vi "Station Get By IP.vi"(8 "error in (no error)":errorcluster, 10 "IP or Name (\"\")":string, 11 "Connection Refnum":T3) -> (0 "error out":errorcluster, 1 "Instruments on Station":T2[](array[typedef]), 2 "Station Record":T1, 3 "Connection Refnum":T3, 4 "Data Present?":bool, 6 "Stand Alone?":bool)   [LabVIEW 2011]
uses:
  SI.LIB/ODBC/SQL Controls/Connection Refnum.ctl
  Instruments/Instrument Record.ctl
  Station Record.ctl
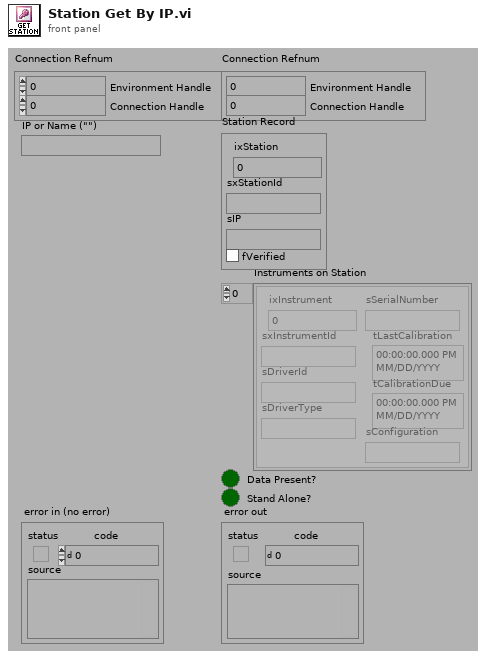
[diagram p1: front panel]
types:
  T1 = typedef "Station Record.ctl" = cluster{"ixStation":i32, "sxStationId":string, "sIP":string, "fVerified":bool}
  T2 = typedef "Instrument Record.ctl" = cluster{"ixInstrument":i32, "sxInstrumentId":string, "sDriverId":string, "sDriverType":string, "sSerialNumber":string, "tLastCalibration":timestamp, "tCalibrationDue":timestamp, "sConfiguration":string}
  T3 = typedef "Connection Refnum.ctl" = cluster{"Environment Handle":i32, "Connection Handle":i32}
  T4 = typedef "Statement Refnum.ctl" = cluster{"Statement Handle":i32, "Parameter Number":u16}
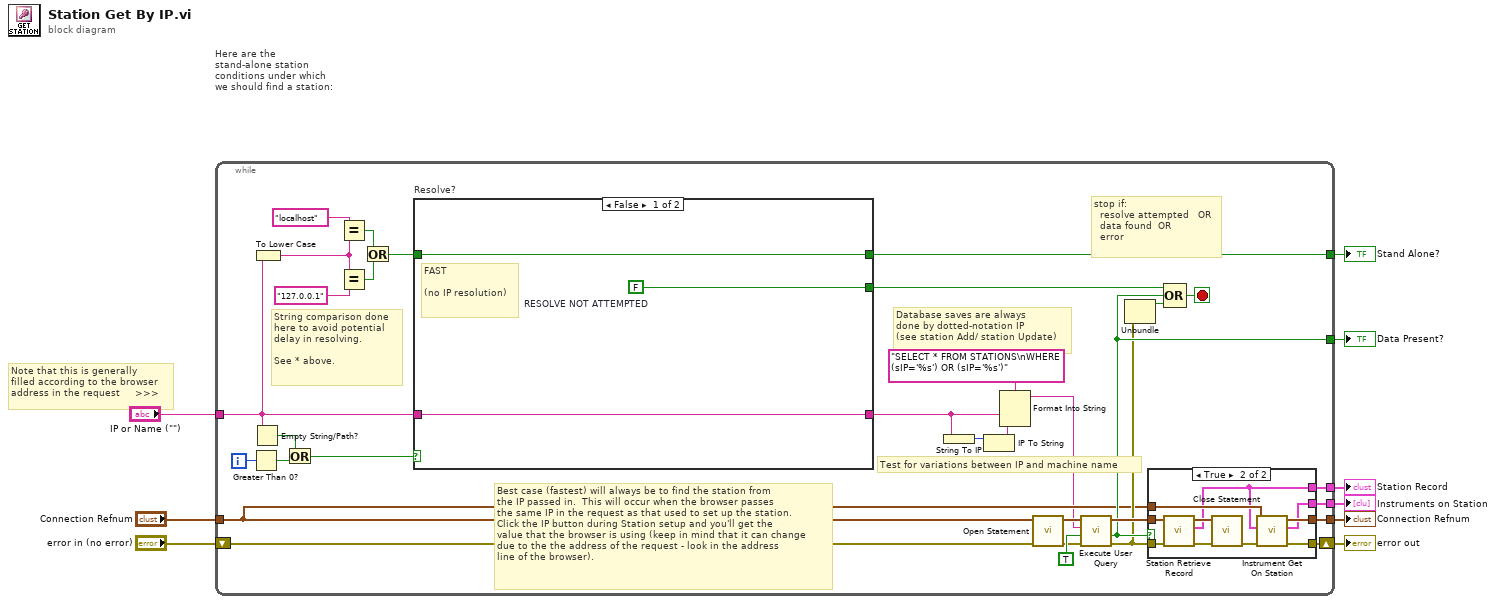
[diagram p0: block diagram]
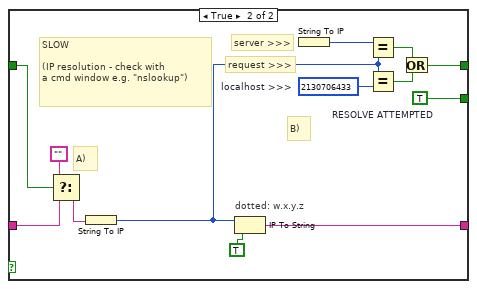
[diagram p2: hidden frame]
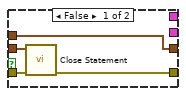
[diagram p3: hidden frame]
diagram:
  # "Note that this is generally\nfilled according to the browser\naddress in the request     >>>"
  n1 = while "Here are the stand-alone station conditions under which we should find a station:\n\n    1) Station saved by \"real\" IP (or domain name);  Request is from 127.0.0.1 (or localhost)\n    2) Station saved by \"127.0.0.1\" or (localhost);  Request from \"real\" IP (or domain name)\n---------------\n0 (fast).  Try query by incoming IP (or Name) without resolving    \n1 (slow).  If not found, try resolving incoming IP, then query.\n                a)  if incoming is \"localhost\" or \"127.0.0.1\" then force to empty \"\" as we've\n                     already looked for these in the first pass;\n                b) if incoming is NOT localhost IP, try to resolve, and compare resolved IP (numeric)\n                    with the server's IP to get \"stand-alone\" status." {
    tunnel: [w38] -> w9
    tunnel: "Connection Refnum" -> [w26]
    tunnel: "IP or Name (\"\")" -> [w17]
    tunnel: [w25] -> w5
    shift-right: [w27] -> w6
    shift-left: "error in (no error)" -> [w33]
    tunnel: [w13] -> w7
    tunnel: [w12] -> w4
    tunnel: [w11] -> w3
    i -> [w39]
    stop <- w37 stop-if-true
    # "Test for variations between IP and machine name"
    # "String comparison done\nhere to avoid potential\ndelay in resolving. \n\nSee * above."
    # "Database saves are always\ndone by dotted-notation IP\n(see station Add/ station Update)"
    # "Best case (fastest) will always be to find the station from\nthe IP passed in.  This will occur when the browser passes\nthe same IP in the request as that used to set up the station.\nClick the IP button during Station setup and you'll get the\nvalue that the browser is using (keep in mind that it can change\ndue to the the address of the request - look in the address\nline of the browser)."
    # "stop if:\n  resolve attempted   OR\n  data found  OR\n  error"
    n2 = Greater Than 0?(x=w39) -> (x > 0?=w29:bool)
    n3 = Empty String/Path?(string/path=w17) -> (empty?=w30:bool)
    n4 = To Lower Case(string=w17) -> (all lower case string=w18:string)
    n5 = Or(x=w30, y=w29) -> (x .or. y?=w28:bool)
    n6 = Equal?(x="localhost", y=w18) -> (x = y?=w21:bool)
    n7 = Equal?(x=w18, y="127.0.0.1") -> (x = y?=w22:bool)
    n8 = Or(x=w21, y=w22) -> (x .or. y?=w16:bool)
    n9 = case "Resolve?" shown="False" w28 {
      tunnel: [w43 w57] -> w10
      tunnel: w17 -> [w43 w54]
      tunnel: [w44 w45] -> w31
      tunnel: [w42 w46] -> w13
      tunnel: w16 -> [w42 w55]
      frame False {
        w44 = FALSE  # RESOLVE NOT ATTEMPTED
        # "FAST\n\n(no IP resolution)"
      }
      frame True {
        w45 = TRUE  # RESOLVE ATTEMPTED
        w49 = u32 2130706433  # localhost >>>
        # "B)"
        # "request >>>"
        # "server >>>"
        # "A)"
        # "SLOW\n\n(IP resolution - check with\na cmd window e.g. \"nslookup\")"
        # "dotted: w.x.y.z"
        n10 = Select(t="", s=w55, f=w54) -> (s? t:f=w53:string)
        n11 = String To IP(1:w53) -> (0:w47:u32)
        n12 = IP To String(1:TRUE, 2:w47) -> (0:w57:string)
        n13 = String To IP() -> (0:w51:u32)  [unwired: 1 out]
        n14 = Equal?(x=w51, y=w47) -> (x = y?=w50:bool)
        n15 = Equal?(x=w47, y=w49) -> (x = y?=w48:bool)
        n16 = Or(x=w50, y=w48) -> (x .or. y?=w46:bool)
      }
    }
    n17 = String To IP(1:w10) -> (0:w15:u32)
    n18 = IP To String(2:w15) -> (0:w14:string)  [unwired: 1 out]
    n19 = Format Into String(format string="SELECT * FROM STATIONS\nWHERE (sIP='%s') OR (sIP='%s')" ("User Query"), w10, w14) -> (resulting string=w23:string)  [unwired: 2 in, 1 out]
    n20 = call "Open Statement.vi"("error in (no error)"=w33, "Connection Refnum"=w26) -> ("error out"=w32:errorcluster, "Statement Refnum"=w34:T4)  [unwired: 4 out]
    n21 = call "Execute User Query.vi"("error in (no error)"=w32, "Return Data? (f)"=TRUE, "User Query"=w23, "Statement Refnum"=w34) -> ("error out"=w36:errorcluster, "Data Present?"=w38:bool, "Statement Refnum"=w41:T4)  [unwired: 1 out]
    n22 = Unbundle(w36) -> ("status"=w35:bool)  [unwired: 2 out]
    n23 = case shown="True" w38 {
      tunnel: w36 -> [w61 w71]
      tunnel: w41 -> [w60 w70]
      tunnel: [w59 w66] -> w27
      tunnel: w26 -> [w58 w65]
      tunnel: [w58 w64] -> w25
      tunnel: [_ w63] -> w12
      tunnel: [_ w62] -> w11
      frame False {
        n24 = call "Close Statement.vi"("error in (no error)"=w61, "Statement Refnum"=w60) -> ("error out"=w59:errorcluster)  [unwired: 5 out]
      }
      frame True {
        n25 = call "Station Retrieve Record.vi"("error in (no error)"=w71, "Statement Refnum"=w70) -> ("error out"=w68:errorcluster, "Station Record"=w63:T1, "Statement Refnum"=w69:T4)  [unwired: 7 out]
        n26 = call "Close Statement.vi"("error in (no error)"=w68, "Statement Refnum"=w69) -> ("error out"=w67:errorcluster)  [unwired: 5 out]
        n27 = call "Instrument Get On Station.vi"("error in (no error)"=w67, "Station Record"=w63, "Connection Refnum"=w65) -> ("error out"=w66:errorcluster, "Instruments on Station"=w62:T2[], "Connection Refnum"=w64:T3)  [unwired: 6 out]
      }
    }
    n28 = Compound Arithmetic op=OR(w31, w38, w35) -> (w37:bool)
  }
  "error out" <- w6
  "Data Present?" <- w9
  "Connection Refnum" <- w5
  "Stand Alone?" <- w7
  "Instruments on Station" <- w3
  "Station Record" <- w4
